vi "Test.Maui 2.0.Initialize.Scarce.Rings.Ring 3.vi"(8 "error in":errorcluster) -> (0 "error out":errorcluster)   [LabVIEW 2020]
uses:
  Maui 2.0/Maui 2.0.lvclass
  C:/Program Files (x86)/National Instruments/LabVIEW 2020/vi.lib/JKI/JKI SMO/SMO/SMO.lvclass
  Helper/Test Helper 1/Test Helper 1.lvclass
  <vilib>/addons/_JKI Toolkits/Caraya/classes/Assert/Assert Equal Value_Variant.vi
  <vilib>/JKI/JKI SMO/SMO/SMO.lvclass
  <vilib>/addons/_JKI Toolkits/Caraya/classes/Assert/Assert.lvclass
  <vilib>/addons/_JKI Toolkits/Caraya/classes/Test/Test.lvclass
panel:
  in  "Ring 3":u16(ring) items=["Test Helper 1", "None"]
  in  "Ring 2":u16(ring) items=["Test Helper 1", "None"]
  in  "Ring":u16(ring) items=["Test Helper 1", "None"]
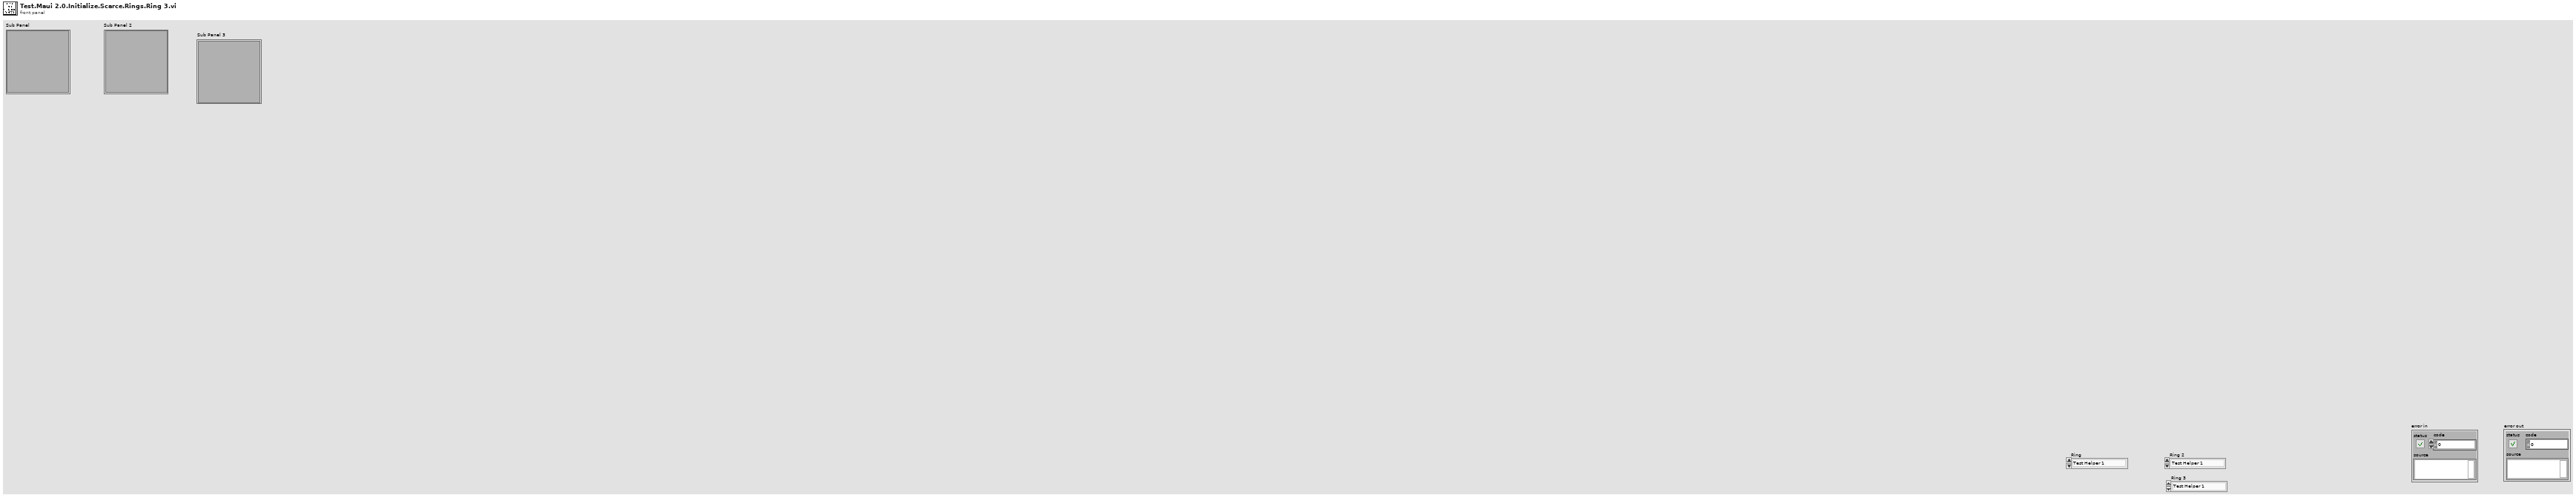
[diagram p1: front panel]
types:
  T1 = cluster{"Ring 3":refnum<vi>, "Sub Panel 3":refnum<vi>}
  T2 = cluster{"Ring":refnum<vi>, "Sub Panel":refnum<vi>}
  T3 = cluster{"Ring 2":refnum<vi>, "Sub Panel 2":refnum<vi>}
  T4 = cluster{"Ring 3":refnum<vi>, "Sub Panel 3":refnum<vi>}[]
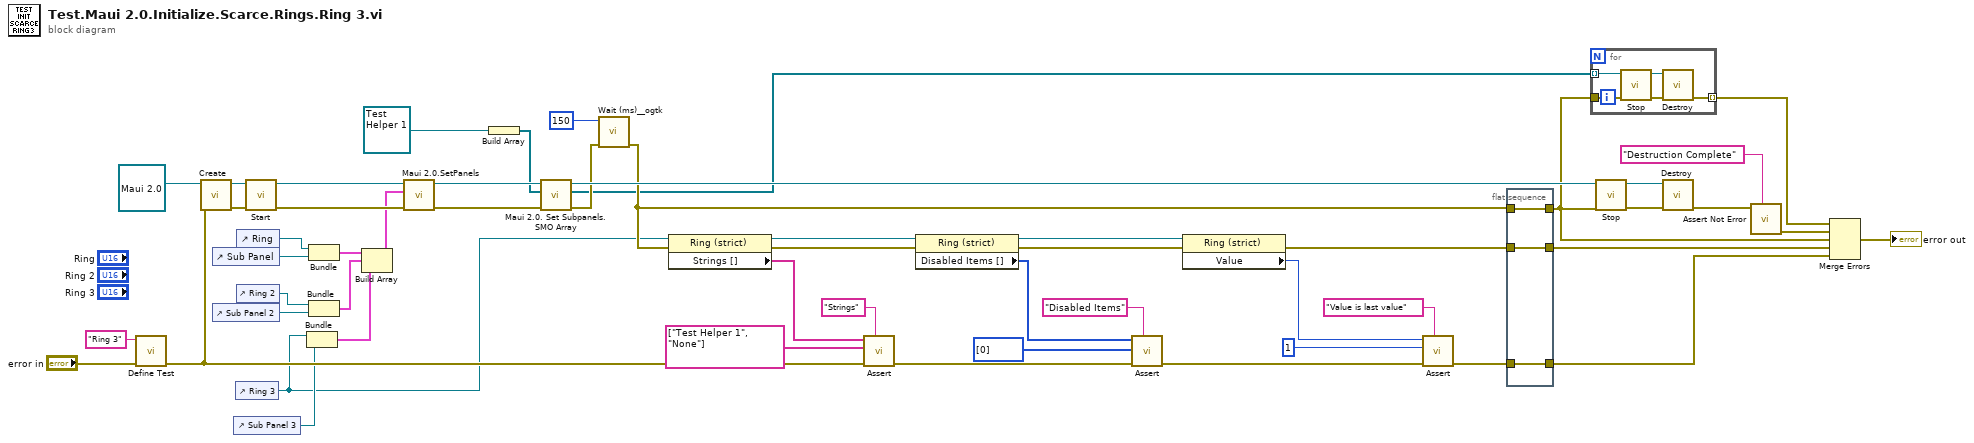
[diagram p0: block diagram]
diagram:
  n1 = call <vilib>:"Define Test.vi"("error in (no error)"="error in", "Label (VI Title)"="Ring 3") -> ("error out"=w30:errorcluster)  [unwired: 9 in]
  n2 = call <vilib>:"Create.vi"("error in (no error)"=w30, "SMO"=refnum<class "Maui 2.0.lvclass"> refnum ("Maui 2.0 in")) -> ("error out"=w54:errorcluster, "SMO out"=w47:refnum<class "Maui 2.0.lvclass">)  [unwired: 7 in, 1 out]
  n3 = control-ref of="Sub Panel"() -> (w51:refnum<vi>)
  n4 = control-ref of="Sub Panel 2"() -> (w50:refnum<vi>)
  n5 = control-ref of="Sub Panel 3"() -> (w4:refnum<vi>)
  n6 = control-ref of="Ring 3"() -> (w3:refnum<vi>)
  n7 = control-ref of="Ring"() -> (w40:refnum<vi>)
  n8 = control-ref of="Ring 2"() -> (w6:refnum<vi>)
  n9 = call <vilib>:"Start.vi"("error in (no error)"=w54, "SMO"=w47) -> ("error out"=w53:errorcluster, "SMO out"=w45:refnum<class "Maui 2.0.lvclass">)  [unwired: 8 in]
  n10 = Bundle("Ring 3"=w3, "Sub Panel 3"=w4) -> (w2:T1)  [unwired: 1 in]
  n11 = Bundle("Ring"=w40, "Sub Panel"=w51) -> (w49:T2)  [unwired: 1 in]
  n12 = Bundle("Ring 2"=w6, "Sub Panel 2"=w50) -> (w48:T3)  [unwired: 1 in]
  n13 = Build Array(w49, w48, w2) -> (w41:T4)
  n14 = call "Maui 2.0.SetPanels.vi"("error in (no error)"=w53, "Set Panels"=w41, "Maui 2.0"=w45) -> ("error out"=w52:errorcluster, "Maui 2.0 out"=w44:refnum<class "Maui 2.0.lvclass">)  [unwired: 7 in]
  n15 = Build Array(refnum<class "Test Helper 1.lvclass"> refnum ("Test Helper 1.lvclass")) -> (w42:refnum<class "Test Helper 1.lvclass">[])
  n16 = call-dynamic "Maui 2.0. Set Subpanels.SMO Array.vi"("error in (no error)"=w52, "Subpanels in"=w42, "Maui 2.0 in"=w44) -> ("error out"=w15:errorcluster, "Subpanels Out"=w12:refnum<class "SMO.lvclass">[], "Maui 2.0 out"=w25:refnum<class "Maui 2.0.lvclass">)  [unwired: 6 in]
  n17 = call <userlib>:"Wait (ms)__ogtk.vi"("error in (no error)"=w15, "milliseconds to wait"=u32 150) -> ("error out"=w14:errorcluster)  [unwired: 8 in, 1 out]
  n18 = property on="Property Node" class="Ring (strict)"(reference=w3, error in=w14) -> (reference out=w34:refnum<vi>, error out=w28:errorcluster, "Strings []"=w38:string[])
  n19 = call-poly <vilib>:"Assert.vi"("Label"="Strings", "error in (no error)"=w30, "Y"=string[] ["Test Helper 1", "None"], "X"=w38) -> ("error out"=w29:errorcluster)  [unwired: 7 in]
  n20 = property on="Property Node" class="Ring (strict)"(reference=w34, error in=w28) -> (reference out=w32:refnum<vi>, error out=w27:errorcluster, "Disabled Items []"=w9:i32[])
  n21 = call-poly <vilib>:"Assert.vi"("Label"="Disabled Items", "error in (no error)"=w29, "Y"=i32[] [0] ("Disabled Items []"), "X"=w9) -> ("error out"=w1:errorcluster)  [unwired: 7 in]
  n22 = property on="Property Node" class="Ring (strict)"(reference=w32, error in=w27) -> (error out=w19:errorcluster, "Value"=w26:u16)  [unwired: 1 out]
  n23 = call-poly <vilib>:"Assert.vi"("Label"="Value is last value", "error in (no error)"=w1, "Y"=u16 1 ("Value"), "X"=w26) -> ("error out"=w18:errorcluster)  [unwired: 7 in]
  n24 = flat-sequence {
    tunnel: w14 -> [w57]
    tunnel: w19 -> [w56]
    tunnel: w18 -> [w55]
    tunnel: [w57] -> w10
    tunnel: [w56] -> w17
    tunnel: [w55] -> w16
    frame #0 {
    }
  }
  n25 = for {
    tunnel: w12 -> [w61] mode=indexing
    tunnel: w10 -> [w60]
    tunnel: [w58] -> w11 mode=indexing
    n26 = call <vilib>:"Stop.vi"("error in (no error)"=w60, "SMO"=w61) -> ("error out"=w59:errorcluster, "SMO out"=w62:refnum<class "SMO.lvclass">)  [unwired: 8 in]
    n27 = call <vilib>:"Destroy.vi"("error in (no error)"=w59, "SMO"=w62) -> ("error out"=w58:errorcluster)  [unwired: 9 in]
  }
  n28 = call <vilib>:"Stop.vi"("error in (no error)"=w10, "SMO"=w25) -> ("error out"=w23:errorcluster, "SMO out"=w24:refnum<class "Maui 2.0.lvclass">)  [unwired: 8 in]
  n29 = call <vilib>:"Destroy.vi"("error in (no error)"=w23, "SMO"=w24) -> ("error out"=w22:errorcluster)  [unwired: 9 in]
  n30 = call <vilib>:"Assert Not Error.vi"("Label"="Destruction Complete", "Not Error?"=w22) -> ("error out"=w20:errorcluster)  [unwired: 9 in]
  n31 = Merge Errors(w11, w20, w10, w17, w16) -> (→"error out":errorcluster)
